vi "autotronica final.vi"() -> ()   [LabVIEW 2026]
uses:
  <vilib>/MakerHub/LINX/Public/Peripherals/Digital/Digital Read 1 Chan.vi
  <vilib>/MakerHub/LINX/Public/Peripherals/Analog/Analog Read 1 Chan.vi
  <vilib>/MakerHub/LINX/Public/Peripherals/Digital/Digital Read N Chans.vi
  <vilib>/MakerHub/LINX/Public/Peripherals/Analog/Analog Read N Chans.vi
  <vilib>/MakerHub/LINX/Private/Local IO/LinxDigitalRead.vi
  <vilib>/MakerHub/LINX/Public/Utilities/Check Channel.vi
  <vilib>/MakerHub/LINX/Private/Local IO/LinxAnalogRead.vi
  <vilib>/MakerHub/LINX/Public/Utilities/Open Serial.vi
  <vilib>/MakerHub/LINX/Private/Utilties/Generate Error.vi
  <vilib>/express/express shared/transition.llb/Dynamic To Waveform Array.vi
  <vilib>/express/express signal manip/GetorSetDDTAttributes/Set DDT Attributes/SetT0.vi
  <vilib>/express/express shared/transition.llb/Waveform Array To Dynamic.vi
  <vilib>/express/express signal manip/GetorSetDDTAttributes/Set DDT Attributes/Set DDT Properties.xnode
  <vilib>/express/express arith-compare/Formula/XNode/ExpressFormulaBlockNode.xnode
  <vilib>/MakerHub/LINX/LMH-LINX.lvlib
panel:
  out "Waveform Chart":dynamicdata(graph)
  in  "stop":bool
  out "Numeric 6":dbl
  out "Farhenheit":dbl
  out "kelvin":dbl
  out "GRADOS CENTIGRADOS":dbl
  out "Numeric 2":dbl
  out "Numeric":dbl
  out "CARGA DE BATERIA":u8(slide) scale=0.0..100.0
  out "TEMPERATURA":dbl(slide) scale=0.0..100.0
  out "RPM´S":dbl(knob) scale=0.0..8000.0
  in  "Serial Port":refnum<visa-resource-name>="N/A"
  out "PRESION DE FRENADO":dbl(knob) scale=0.0..500.0
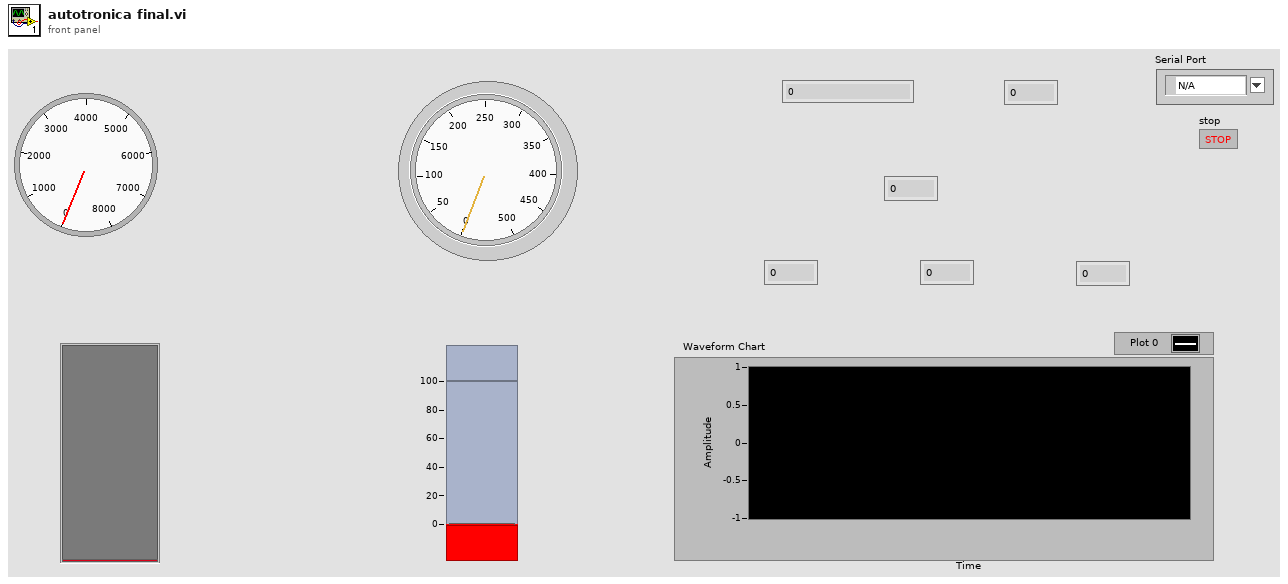
[diagram p1: front panel]
types:
  T1 = typedef "LMH-LINX.lvlib/LINX Ref.ctl" = cluster{"IO":T2, "Interface":T3, "LINX Device Config":T4}
  T2 = typedef "LMH-LINX.lvlib/Platform.ctl" = enum16{"Remote", "Local"}
  T3 = typedef "LMH-LINX.lvlib/Interface.ctl" = enum16{"Serial", "TCP"}
  T4 = typedef "LMH-LINX.lvlib/Device.lvlib/LINX Device Config.ctl" = cluster{"Interface":T3, "COM Port":refnum<visa-resource-name>, "TCP Configuration":T5, "Device Family":u8, "Device ID":u8, "Device Name":string, "TCP Ref":refnum<k5>, "Channels":T6}
  T5 = typedef "LMH-LINX.lvlib/Device.lvlib/TCP Config.ctl" = cluster{"IP Address":string, "Port":u16}
  T6 = typedef "LMH-LINX.lvlib/Channels.ctl" = cluster{"DI":u8[], "DO":u8[], "AI":u8[], "AO":u8[], "PWM":u8[], "QE":u8[], "UART":u8[], "I2C 2":u8[], "SPI":u8[], "CAN":u8[], "Servo":u8[], "AI Ref (V)":dbl, "AI Resolution (Bits)":u8, "AO Ref (V)":dbl, "AO Resolution (Bits)":u8}
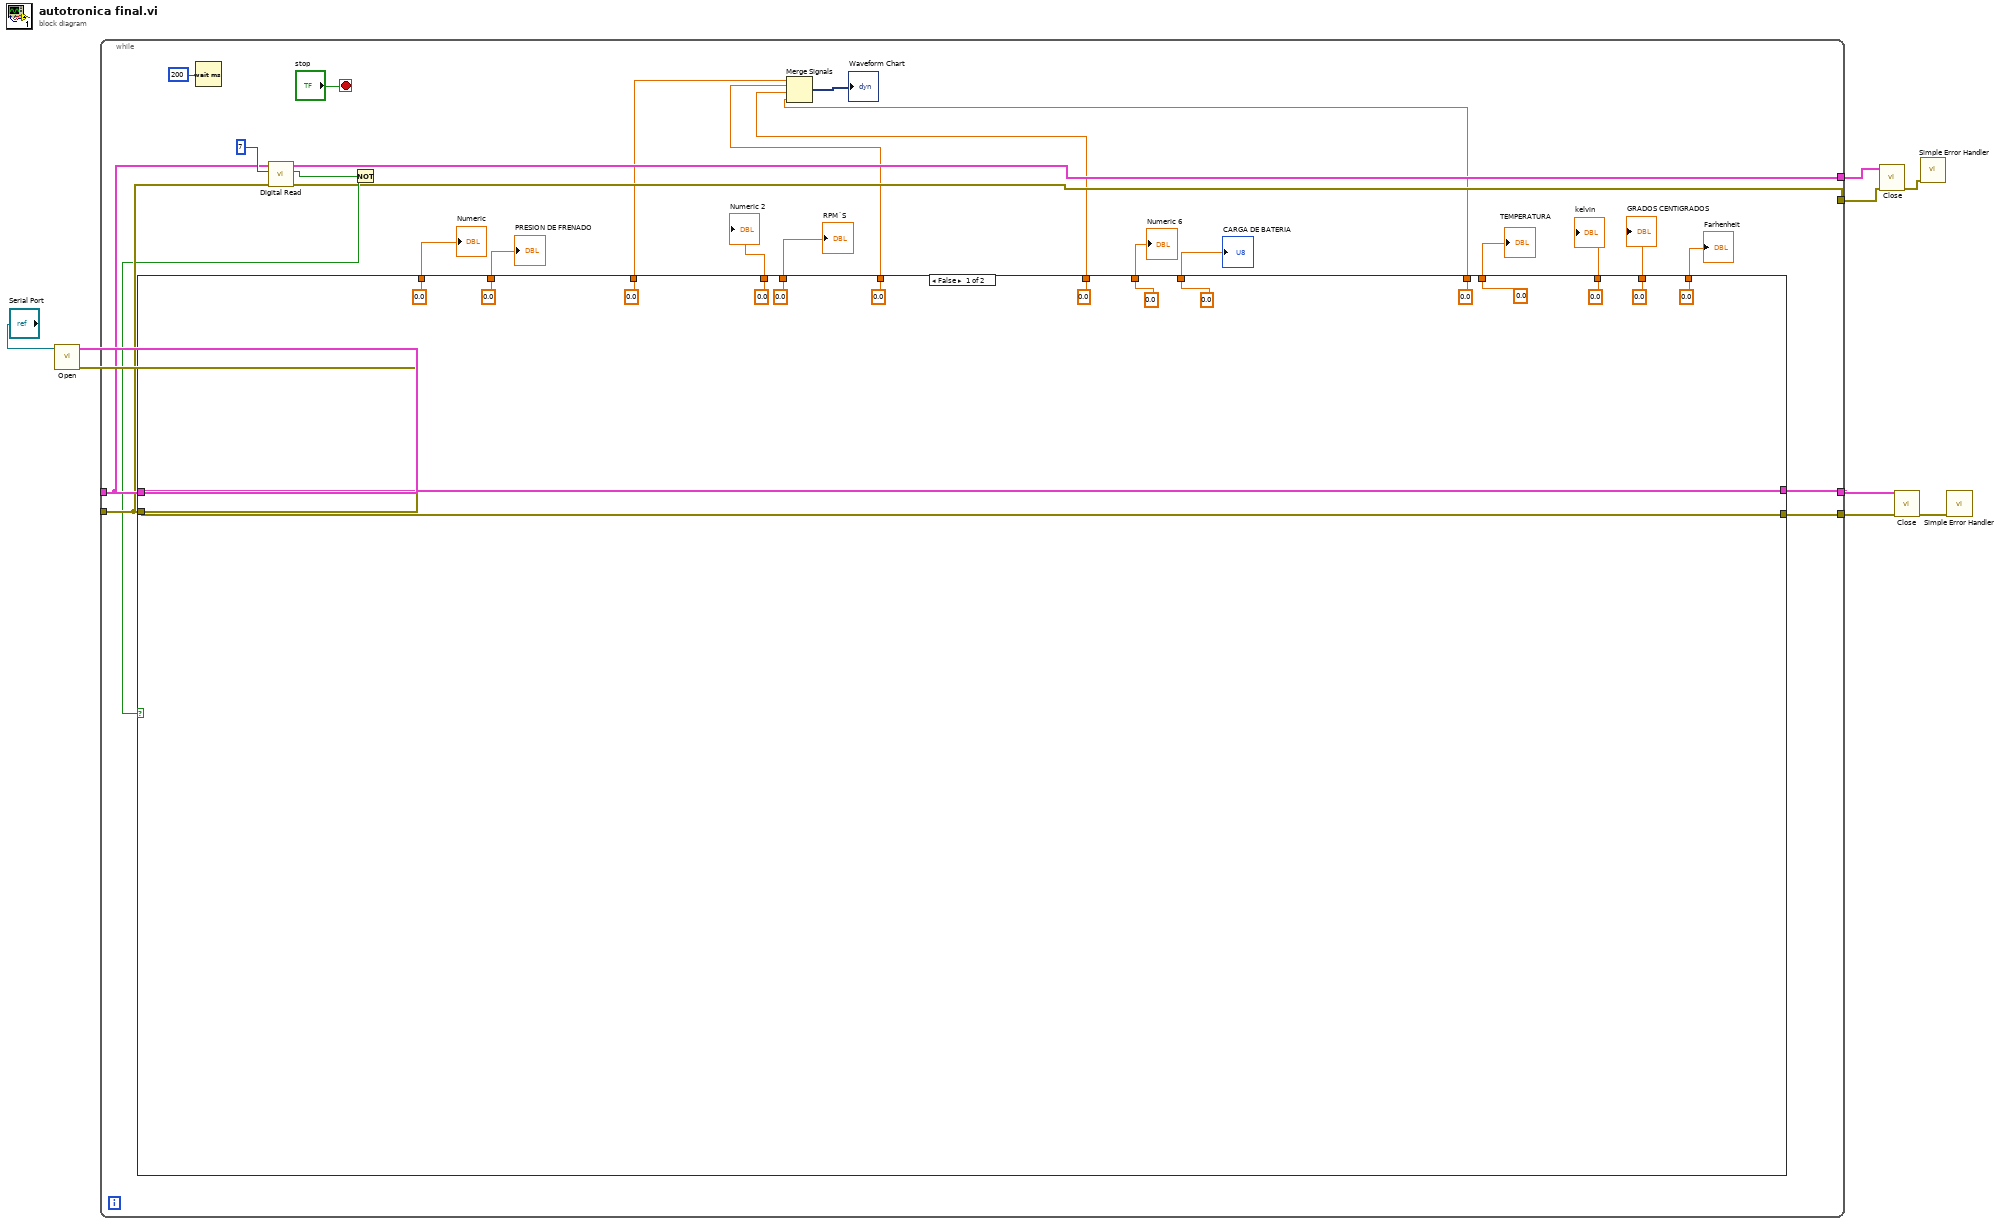
[diagram p0: block diagram]
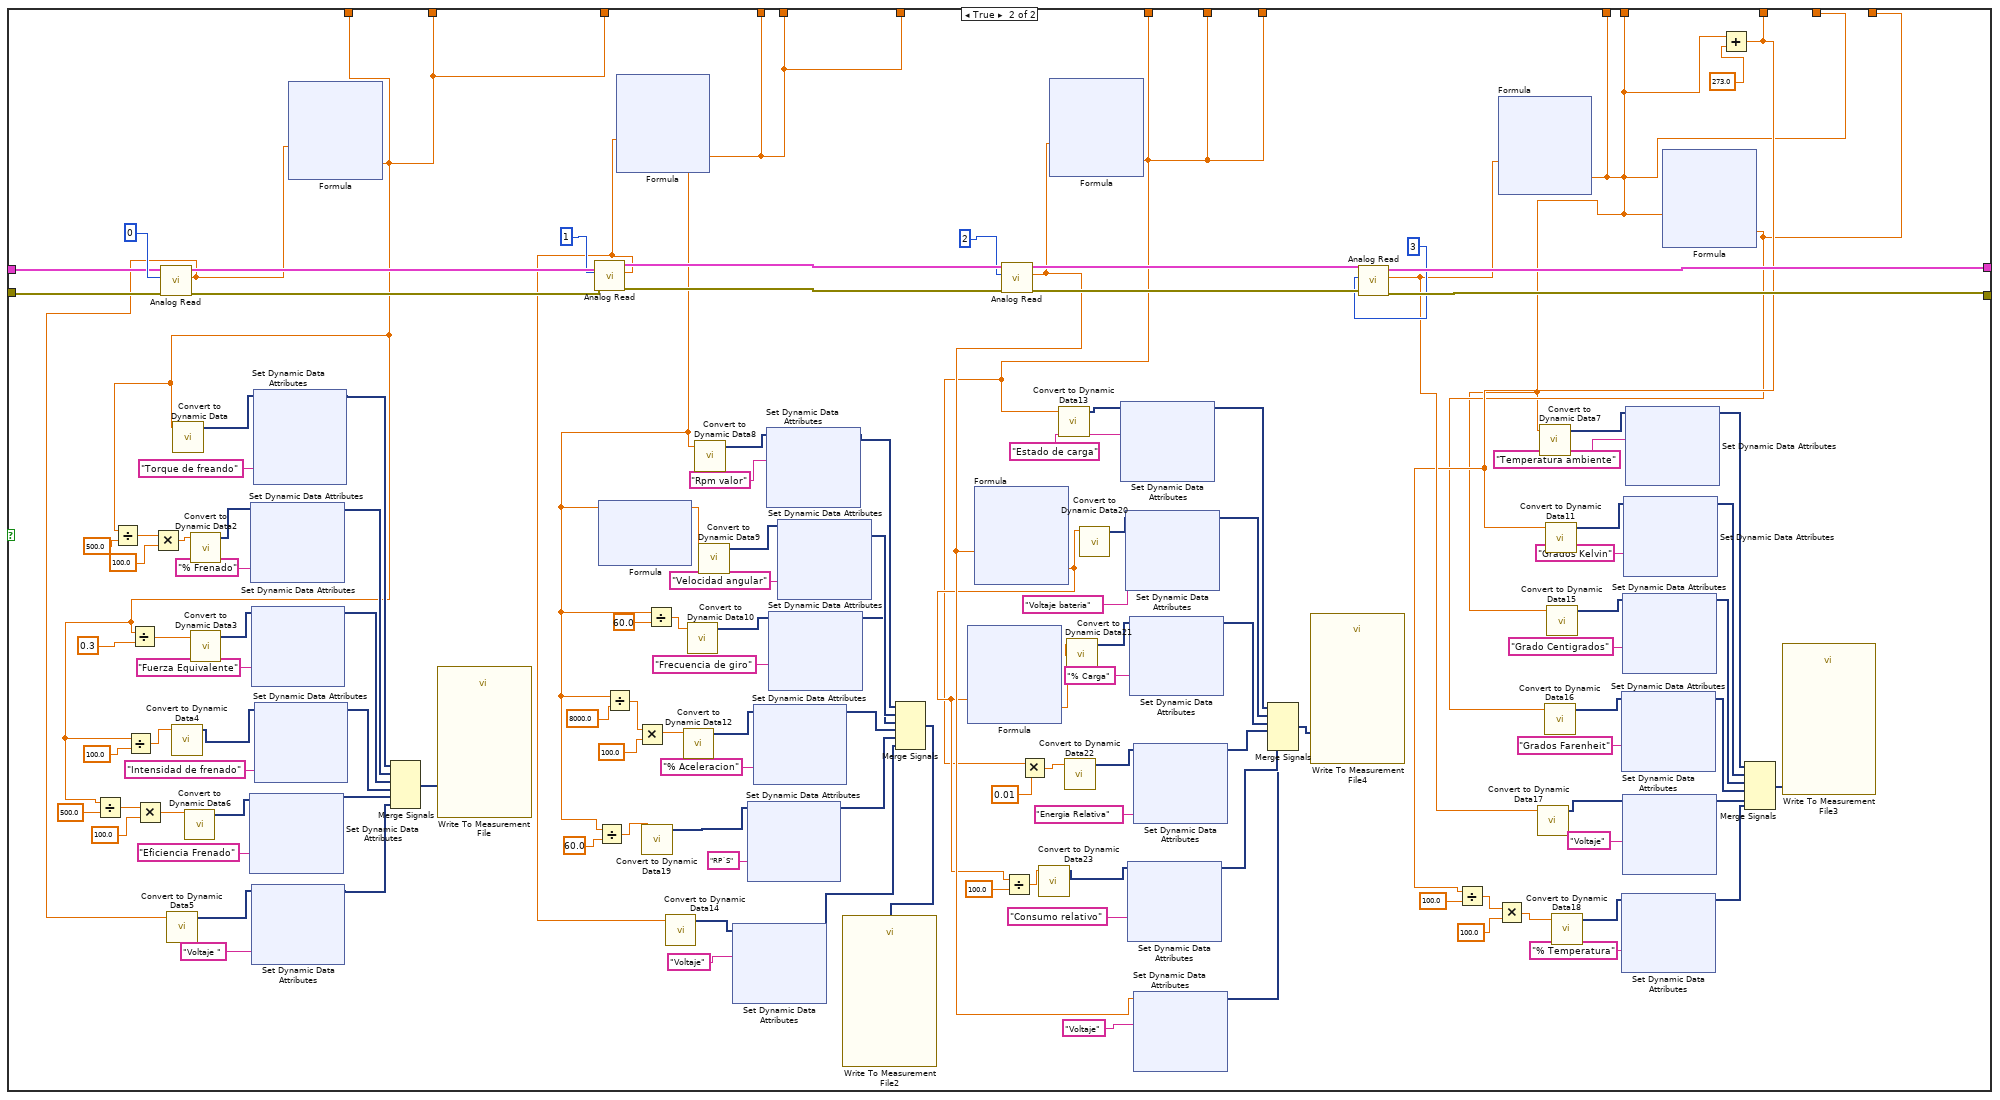
[diagram p2: hidden frame]
diagram:
  n1 = call-poly <vilib>:"Open.vi"("Serial Port"="Serial Port") -> ("Error Out"=w7:errorcluster, "LINX Resource"=w8:T1)  [unwired: 8 in, 1 out]
  n2 = while {
    tunnel: w8 -> [w31]
    tunnel: w7 -> [w30]
    tunnel: [w35] -> w6
    tunnel: [w34] -> w5
    tunnel: [w27] -> w2
    tunnel: [w26] -> w1
    stop <- "stop" stop-if-true
    n3 = Wait (ms)(milliseconds to wait=u32 200) -> ()  [unwired: 1 out]
    n4 = call-poly <vilib>:"Digital Read.vi"("Error In"=w30, "DI Channel"=u8 7, "LINX Resource"=w31) -> ("Error Out"=w26:errorcluster, "DI Value"=w29:bool, "LINX Resource"=w27:T1)  [unwired: 6 in]
    n5 = Not(x=w29) -> (.not. x?=w28:bool)
    n6 = case shown="False" w28 {
      tunnel: w31 -> [w41 w181]
      tunnel: w30 -> [w40 w180]
      tunnel: [w41 w173] -> w35
      tunnel: [w40 w172] -> w34
      tunnel: [0.0 ("Result") w56] -> w24
      tunnel: [0.0 ("Result") w55] -> w23
      tunnel: [0.0 ("Result") w54] -> w22
      tunnel: [0.0 w74] -> w21
      tunnel: [0.0 ("Result") w53] -> w20
      tunnel: [0.0 ("Result") w73] -> w19
      tunnel: [0.0 ("Result") w56] -> w18
      tunnel: [0.0 ("Result") w55] -> w17
      tunnel: [0.0 ("Result") w54] -> w16
      tunnel: [0.0 ("Result") w53] -> w15
      tunnel: [0.0 ("Result") w56] -> w13
      tunnel: [0.0 ("Result") w55] -> w12
      tunnel: [0.0 ("Result") w54] -> w11
      tunnel: [0.0 ("Result") w53] -> w10
      frame False {
      }
      frame True {
        n7 = call-poly <vilib>:"Analog Read.vi"("Error In"=w180, "Analog Channel"=u8 0, "LINX Resource"=w181) -> ("Error Out"=w178:errorcluster, "Voltage"=w71:dbl, "LINX Resource"=w179:T1)  [unwired: 5 in, 1 out]
        n8 = call "Convert to Dynamic Data5"("Double"=w71) -> ("Dynamic Data Type"=w147:dynamicdata)  [unwired: 3 in]
        n9 = xnode "Set Dynamic Data Attributes"("Signals In"=w147, "Signal Name"="Voltaje ") -> ("Signals Out"=w146:dynamicdata)  [unwired: 2 in, 1 out]
        n10 = xnode "Formula"("X1"=w71) -> ("Result"=w56:dbl)  [unwired: 1 in, 1 out]
        n11 = Divide(x=w56, y=500.0) -> (x/y=w60:dbl)
        n12 = Divide(x=w56, y=500.0) -> (x/y=w162:dbl)
        n13 = Divide(x=w56, y=100.0) -> (x/y=w69:dbl)
        n14 = Divide(x=w56, y=0.3) -> (x/y=w155:dbl)
        n15 = Multiply(x=w60, y=100.0) -> (x*y=w58:dbl)
        n16 = Multiply(x=w162, y=100.0) -> (x*y=w161:dbl)
        n17 = call "Convert to Dynamic Data4"("Double"=w69) -> ("Dynamic Data Type"=w72:dynamicdata)  [unwired: 3 in]
        n18 = call "Convert to Dynamic Data"("Double"=w56) -> ("Dynamic Data Type"=w166:dynamicdata)  [unwired: 3 in]
        n19 = call "Convert to Dynamic Data6"("Double"=w58) -> ("Dynamic Data Type"=w57:dynamicdata)  [unwired: 3 in]
        n20 = call "Convert to Dynamic Data2"("Double"=w161) -> ("Dynamic Data Type"=w160:dynamicdata)  [unwired: 3 in]
        n21 = call "Convert to Dynamic Data3"("Double"=w155) -> ("Dynamic Data Type"=w154:dynamicdata)  [unwired: 3 in]
        n22 = xnode "Set Dynamic Data Attributes"("Signals In"=w57, "Signal Name"="Eficiencia Frenado") -> ("Signals Out"=w150:dynamicdata)  [unwired: 2 in, 1 out]
        n23 = xnode "Set Dynamic Data Attributes"("Signals In"=w160, "Signal Name"="% Frenado") -> ("Signals Out"=w158:dynamicdata)  [unwired: 2 in, 1 out]
        n24 = xnode "Set Dynamic Data Attributes"("Signals In"=w154, "Signal Name"="Fuerza Equivalente") -> ("Signals Out"=w153:dynamicdata)  [unwired: 2 in, 1 out]
        n25 = xnode "Set Dynamic Data Attributes"("Signal Name"="Torque de freando", "Signals In"=w166) -> ("Signals Out"=w165:dynamicdata)  [unwired: 2 in, 1 out]
        n26 = xnode "Set Dynamic Data Attributes"("Signals In"=w72, "Signal Name"="Intensidad de frenado") -> ("Signals Out"=w151:dynamicdata)  [unwired: 2 in, 1 out]
        n27 = Merge Signals(w165, w158, w153, w151, w150, w146) -> (w159:dynamicdata)
        n28 = call "Write To Measurement File"("Signals"=w159) -> ()  [unwired: 16 in, 3 out]
        n29 = call-poly <vilib>:"Analog Read.vi"("Error In"=w178, "Analog Channel"=u8 1, "LINX Resource"=w179) -> ("Error Out"=w176:errorcluster, "Voltage"=w124:dbl, "LINX Resource"=w177:T1)  [unwired: 5 in, 1 out]
        n30 = xnode "Formula"("X1"=w124) -> ("Result"=w55:dbl)  [unwired: 1 in, 1 out]
        n31 = Divide(x=w55, y=60.0) -> (x/y=w66:dbl)
        n32 = xnode "Formula"("X1"=w55) -> ("Result"=w140:dbl)  [unwired: 1 in, 1 out]
        n33 = Divide(x=w55, y=8000.0) -> (x/y=w130:dbl)
        n34 = Multiply(x=w130, y=100.0) -> (x*y=w129:dbl)
        n35 = call "Convert to Dynamic Data19"("Double"=w66) -> ("Dynamic Data Type"=w68:dynamicdata)  [unwired: 3 in]
        n36 = Divide(x=w55, y=60.0) -> (x/y=w135:dbl)
        n37 = call "Convert to Dynamic Data14"("Double"=w124) -> ("Dynamic Data Type"=w125:dynamicdata)  [unwired: 3 in]
        n38 = call "Convert to Dynamic Data12"("Double"=w129) -> ("Dynamic Data Type"=w128:dynamicdata)  [unwired: 3 in]
        n39 = call "Convert to Dynamic Data10"("Double"=w135) -> ("Dynamic Data Type"=w134:dynamicdata)  [unwired: 3 in]
        n40 = call "Convert to Dynamic Data8"("Double"=w55) -> ("Dynamic Data Type"=w144:dynamicdata)  [unwired: 3 in]
        n41 = call "Convert to Dynamic Data9"("Double"=w140) -> ("Dynamic Data Type"=w139:dynamicdata)  [unwired: 3 in]
        n42 = xnode "Set Dynamic Data Attributes"("Signals In"=w125, "Signal Name"="Voltaje") -> ("Signals Out"=w121:dynamicdata)  [unwired: 2 in, 1 out]
        n43 = xnode "Set Dynamic Data Attributes"("Signals In"=w68, "Signal Name"="RP´S") -> ("Signals Out"=w122:dynamicdata)  [unwired: 2 in, 1 out]
        n44 = xnode "Set Dynamic Data Attributes"("Signals In"=w128, "Signal Name"="% Aceleracion") -> ("Signals Out"=w127:dynamicdata)  [unwired: 2 in, 1 out]
        n45 = xnode "Set Dynamic Data Attributes"("Signals In"=w144, "Signal Name"="Rpm valor") -> ("Signals Out"=w142:dynamicdata)  [unwired: 2 in, 1 out]
        n46 = xnode "Set Dynamic Data Attributes"("Signals In"=w134, "Signal Name"="Frecuencia de giro") -> ("Signals Out"=w133:dynamicdata)  [unwired: 2 in, 1 out]
        n47 = xnode "Set Dynamic Data Attributes"("Signals In"=w139, "Signal Name"="Velocidad angular") -> ("Signals Out"=w138:dynamicdata)  [unwired: 2 in, 1 out]
        n48 = Merge Signals(w142, w138, w133, w127, w122, w121) -> (w52:dynamicdata)
        n49 = call "Write To Measurement File2"("Signals"=w52) -> ()  [unwired: 16 in, 3 out]
        n50 = call-poly <vilib>:"Analog Read.vi"("Error In"=w176, "Analog Channel"=u8 2, "LINX Resource"=w177) -> ("Error Out"=w174:errorcluster, "Voltage"=w92:dbl, "LINX Resource"=w175:T1)  [unwired: 5 in, 1 out]
        n51 = xnode "Formula"("X1"=w92) -> ("Result"=w63:dbl)  [unwired: 1 in, 1 out]
        n52 = xnode "Formula"("X1"=w63) -> ("Result"=w88:dbl)  [unwired: 1 in, 1 out]
        n53 = Divide(x=w63, y=100.0) -> (x/y=w62:dbl)
        n54 = call "Convert to Dynamic Data23"("Double"=w62) -> ("Dynamic Data Type"=w65:dynamicdata)  [unwired: 3 in]
        n55 = xnode "Formula"("X1"=w92) -> ("Result"=w54:dbl)  [unwired: 1 in, 1 out]
        n56 = Multiply(x=w54, y=0.01) -> (x*y=w85:dbl)
        n57 = call "Convert to Dynamic Data13"("Double"=w54) -> ("Dynamic Data Type"=w93:dynamicdata)  [unwired: 3 in]
        n58 = call "Convert to Dynamic Data22"("Double"=w85) -> ("Dynamic Data Type"=w84:dynamicdata)  [unwired: 3 in]
        n59 = call "Convert to Dynamic Data21"("Double"=w88) -> ("Dynamic Data Type"=w87:dynamicdata)  [unwired: 3 in]
        n60 = call "Convert to Dynamic Data20"("Double"=w63) -> ("Dynamic Data Type"=w91:dynamicdata)  [unwired: 3 in]
        n61 = xnode "Set Dynamic Data Attributes"("Signals In"=w93, "Signal Name"="Estado de carga") -> ("Signals Out"=w81:dynamicdata)  [unwired: 2 in, 1 out]
        n62 = xnode "Set Dynamic Data Attributes"("Signals In"=w91, "Signal Name"="Voltaje bateria") -> ("Signals Out"=w79:dynamicdata)  [unwired: 2 in, 1 out]
        n63 = xnode "Set Dynamic Data Attributes"("Signals In"=w65, "Signal Name"="Consumo relativo") -> ("Signals Out"=w76:dynamicdata)  [unwired: 2 in, 1 out]
        n64 = xnode "Set Dynamic Data Attributes"("Signals In"=w87, "Signal Name"="% Carga") -> ("Signals Out"=w78:dynamicdata)  [unwired: 2 in, 1 out]
        n65 = xnode "Set Dynamic Data Attributes"("Signals In"=w84, "Signal Name"="Energia Relativa") -> ("Signals Out"=w77:dynamicdata)  [unwired: 2 in, 1 out]
        n66 = xnode "Set Dynamic Data Attributes"("Signals In"=w92, "Signal Name"="Voltaje") -> ("Signals Out"=w75:dynamicdata)  [unwired: 2 in, 1 out]
        n67 = Merge Signals(w81, w79, w78, w77, w76, w75) -> (w80:dynamicdata)
        n68 = call "Write To Measurement File4"("Signals"=w80) -> ()  [unwired: 16 in, 3 out]
        n69 = call-poly <vilib>:"Analog Read.vi"("Error In"=w174, "Analog Channel"=u8 3, "LINX Resource"=w175) -> ("Error Out"=w172:errorcluster, "Voltage"=w109:dbl, "LINX Resource"=w173:T1)  [unwired: 5 in, 1 out]
        n70 = xnode "Formula"("X1"=w109) -> ("Result"=w53:dbl)  [unwired: 1 in, 1 out]
        n71 = call "Convert to Dynamic Data17"("Double"=w109) -> ("Dynamic Data Type"=w111:dynamicdata)  [unwired: 3 in]
        n72 = call "Convert to Dynamic Data7"("Double"=w53) -> ("Dynamic Data Type"=w115:dynamicdata)  [unwired: 3 in]
        n73 = call "Convert to Dynamic Data15"("Double"=w53) -> ("Dynamic Data Type"=w113:dynamicdata)  [unwired: 3 in]
        n74 = xnode "Set Dynamic Data Attributes"("Signals In"=w113, "Signal Name"="Grado Centigrados") -> ("Signals Out"=w100:dynamicdata)  [unwired: 2 in, 1 out]
        n75 = xnode "Set Dynamic Data Attributes"("Signals In"=w111, "Signal Name"="Voltaje") -> ("Signals Out"=w98:dynamicdata)  [unwired: 2 in, 1 out]
        n76 = xnode "Set Dynamic Data Attributes"("Signals In"=w115, "Signal Name"="Temperatura ambiente") -> ("Signals Out"=w103:dynamicdata)  [unwired: 2 in, 1 out]
        n77 = xnode "Formula"("X1"=w53) -> ("Result"=w73:dbl)  [unwired: 1 in, 1 out]
        n78 = call "Convert to Dynamic Data16"("Double"=w73) -> ("Dynamic Data Type"=w112:dynamicdata)  [unwired: 3 in]
        n79 = xnode "Set Dynamic Data Attributes"("Signals In"=w112, "Signal Name"="Grados Farenheit") -> ("Signals Out"=w99:dynamicdata)  [unwired: 2 in, 1 out]
        n80 = Add(x=w53, y=273.0) -> (x+y=w74:dbl)
        n81 = Divide(x=w74, y=100.0) -> (x/y=w106:dbl)
        n82 = Multiply(x=w106, y=100.0) -> (x*y=w105:dbl)
        n83 = call "Convert to Dynamic Data11"("Double"=w74) -> ("Dynamic Data Type"=w114:dynamicdata)  [unwired: 3 in]
        n84 = call "Convert to Dynamic Data18"("Double"=w105) -> ("Dynamic Data Type"=w104:dynamicdata)  [unwired: 3 in]
        n85 = xnode "Set Dynamic Data Attributes"("Signals In"=w104, "Signal Name"="% Temperatura") -> ("Signals Out"=w97:dynamicdata)  [unwired: 2 in, 1 out]
        n86 = xnode "Set Dynamic Data Attributes"("Signals In"=w114, "Signal Name"="Grados Kelvin") -> ("Signals Out"=w101:dynamicdata)  [unwired: 2 in, 1 out]
        n87 = Merge Signals(w103, w101, w100, w99, w98, w97) -> (w102:dynamicdata)
        n88 = call "Write To Measurement File3"("Signals"=w102) -> ()  [unwired: 16 in, 3 out]
      }
    }
    "Numeric" <- w24
    "Numeric 2" <- w23
    "Numeric 6" <- w22
    "kelvin" <- w21
    "GRADOS CENTIGRADOS" <- w20
    "Farhenheit" <- w19
    "PRESION DE FRENADO" <- w18
    "RPM´S" <- w17
    "CARGA DE BATERIA" <- w16
    "TEMPERATURA" <- w15
    n89 = Merge Signals(w13, w12, w11, w10) -> (→"Waveform Chart":dynamicdata)
  }
  n90 = call <vilib>:"Close.vi"("Error In"=w1, "LINX Resource"=w2) -> ("Error Out"=w3:errorcluster)  [unwired: 9 in]
  n91 = call <vilib>:"Close.vi"("Error In"=w5, "LINX Resource"=w6) -> ("Error Out"=w4:errorcluster)  [unwired: 9 in]
  n92 = call <vilib>:"Simple Error Handler.vi"("error in (no error)"=w3) -> ()  [unwired: 4 in, 5 out]
  n93 = call <vilib>:"Simple Error Handler.vi"("error in (no error)"=w4) -> ()  [unwired: 4 in, 5 out]
